vi "Parse Report File Name.vi"(0 "File name":path, 1 "regular expression":string="^(report([0-9]+))(\\.txt)$") -> (7 "Full file name":path, 8 "Base file name (no extension)":string, 9 "Report number":i32, 10 "Extension":string)   [LabVIEW 2020, in "Mock LC Parser.lvlib"]
doc: "Parses a report file name, returning a duplicate of the full file name, the base file name (name with no extension), the report number, and the file extension. The default regex used is \"^(report([0-9]+))(\\.txt)$\", which will match report file names of the form: report<number>.txt. All return values will be an emtpy string if the file name does not match the report file name regex, which can be used to validate a report file name."
uses:
  Mock LC Parser.lvlib
  <vilib>/regexp/Match Regular Expression.xnode
panel:
  out "after match":string
  out "before match":string
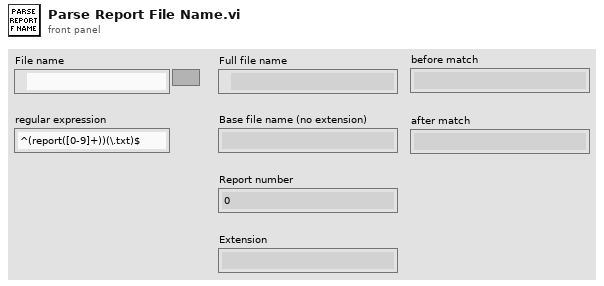
[diagram p1: front panel]
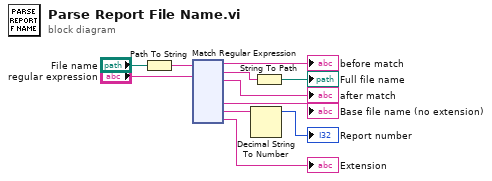
[diagram p0: block diagram]
diagram:
  n1 = Path To String(path="File name") -> (string=w2:string)
  n2 = xnode "Match Regular Expression"("input string"=w2, "regular expression"="regular expression") -> ("before match"=→"before match":string, "whole match"=w8:string, "after match"=→"after match":string, "submatch 1"=→"Base file name (no extension)":string, "submatch 2"=w5:string, "submatch 3"=→"Extension":string)  [unwired: 4 in, 2 out]
  n3 = Decimal String To Number(string=w5) -> (number=→"Report number":i32)  [unwired: 2 in, 1 out]
  n4 = String To Path(string=w8) -> (path=→"Full file name":path)
